vi "Incomplete Analysis.vi"(8 "error constant":errorcluster) -> (0 "error out":errorcluster)   [LabVIEW 2013]
doc: "Use this template to build a simple state machine design pattern. Each state executes code and determines which state to transition to."
uses:
  Analysis Support/Controls/State.ctl
panel:
  out "SPL":dbl
  out "End Flow":dbl format="%0.3f"
  out "Start Flow":dbl format="%0.3f"
  out "Resistance":dbl
  out "Time":dbl
  out "SGP":dbl
  out "selected path":path
  out "Message":string
  in  "Begin":bool
  in  "Exit":bool
  in  "Blank Button":bool
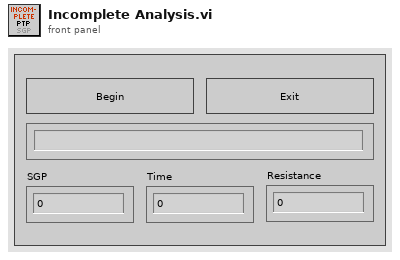
[diagram p1: front panel]
types:
  T1 = typedef "State.ctl" = enum16{"Initialize", "Wait for Event", "Analyze", "Save", "Exit"}
  T2 = enum8{"Enabled", "Disabled", "Disabled and Grayed Out"}
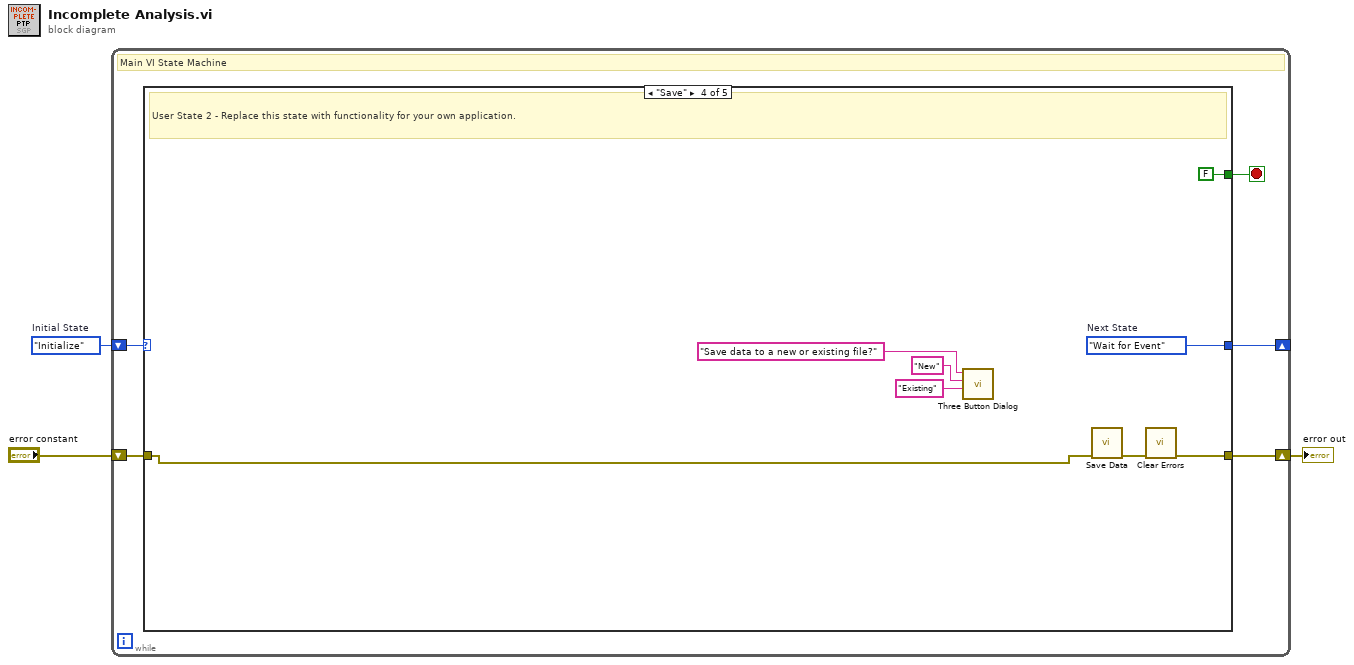
[diagram p0: block diagram]
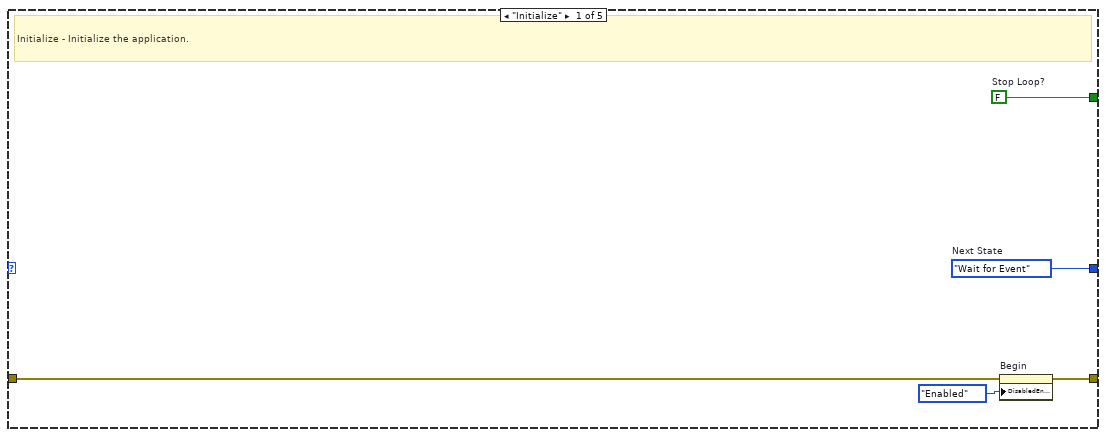
[diagram p2: hidden frame]
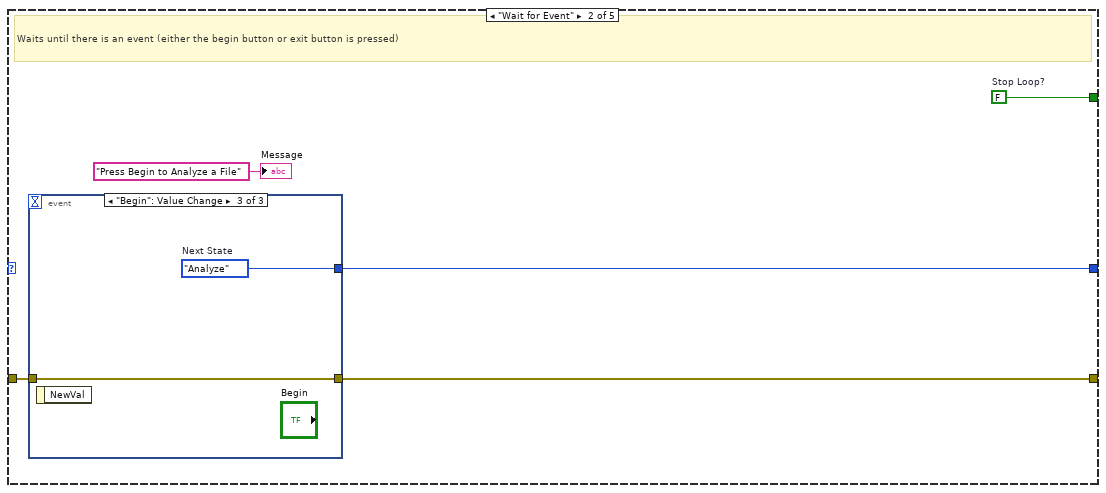
[diagram p3: hidden frame]
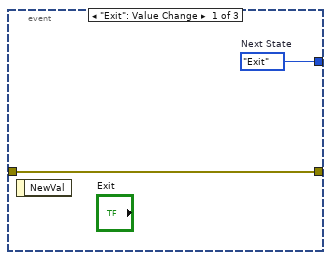
[diagram p4: hidden frame]
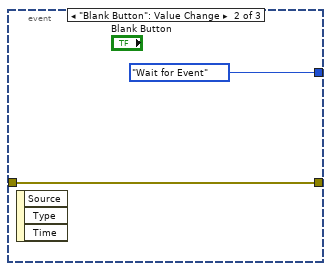
[diagram p5: hidden frame]
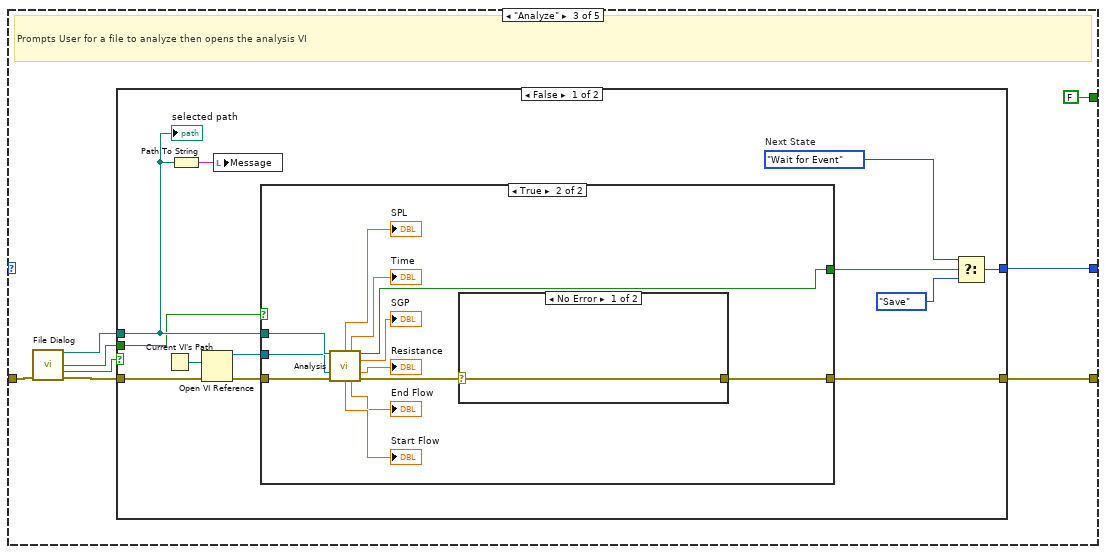
[diagram p6: hidden frame]
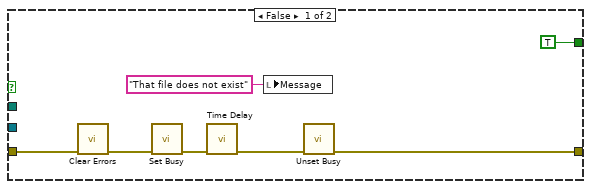
[diagram p7: hidden frame]
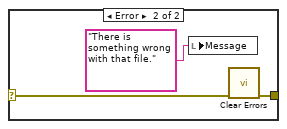
[diagram p8: hidden frame]
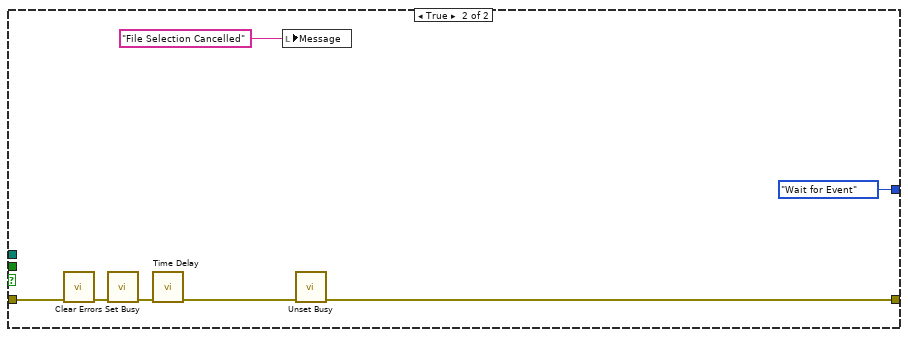
[diagram p9: hidden frame]
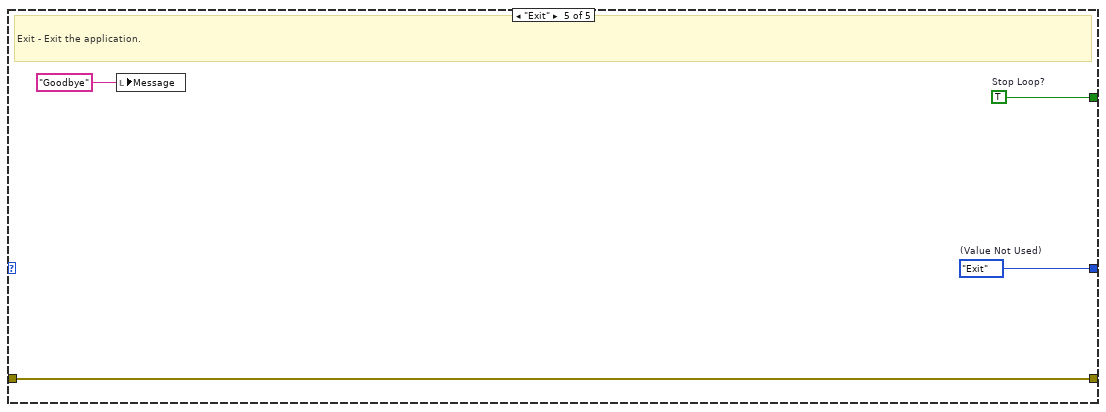
[diagram p10: hidden frame]
diagram:
  w3 = State."Initialize"  # Initial State
  n1 = while {
    shift-right: [w7] -> _
    shift-left: w3 -> [w8]
    shift-right: [w5] -> w1
    shift-left: "error constant" -> [w6]
    stop <- w4 stop-if-true
    # "Main VI State Machine"
    n2 = case shown="\"Save\"" w8 {
      tunnel: [w13 w18 w32 w82 w86] -> w7
      tunnel: [w12 w17 FALSE ("Stop Loop?") FALSE ("Stop Loop?") w85] -> w4
      tunnel: w6 -> [w11 w16 w29 w79 w84]
      tunnel: [w9 w15 w30 w75 w84] -> w5
      frame "Initialize" {
        w12 = FALSE  # Stop Loop?
        w13 = State."Wait for Event"  # Next State
        # "Initialize - Initialize the application."
        n3 = property on="Begin" class="Bool"(error in=w11, "DisabledEnum"=T2."Enabled" ("Disabled")) -> (error out=w9:errorcluster)  [unwired: 1 in, 1 out]
      }
      frame "Wait for Event" {
        w17 = FALSE  # Stop Loop?
        # "Waits until there is an event (either the begin button or exit button is pressed)"
        n4 = event shown="[2] \"Begin\": Value Change" {
          selector: _ -> [_ _ _]
          dyn-events: _ -> [_ _ _]
          timeout: _ -> [_ _ _]
          tunnel: [w20 State."Wait for Event" ("Next State") w24] -> w18
          tunnel: w16 -> [w19 w22 w23]
          tunnel: [w19 w22 w23] -> w15
          event "Exit": Value Change {
            w20 = State."Exit"  # Next State
            n5 = event-data() -> ()  [unwired: 1 in, 1 out]
          }
          event "Blank Button": Value Change {
            n6 = event-data() -> ()  [unwired: 1 in, 3 out]
          }
          event "Begin": Value Change {
            w24 = State."Analyze"  # Next State
            n7 = event-data() -> ()  [unwired: 1 in, 1 out]
          }
        }
        "Message" <- "Press Begin to Analyze a File" ("String")
      }
      frame "Analyze" {
        # "Prompts User for a file to analyze then opens the analysis VI"
        n8 = call "File Dialog"("error in"=w29) -> ("selected path"=w26:path, "exists"=w27:bool, "cancelled"=w25:bool, "error out"=w28:errorcluster)  [unwired: 11 in]
        n9 = case shown="False" w25 {
          tunnel: [w36 State."Wait for Event" ("Next State")] -> w32
          tunnel: [w44 w68] -> w30
          tunnel: w28 -> [w42 w73]
          tunnel: w27 -> [w37 _]
          tunnel: w26 -> [w39 _]
          frame False {
            w35 = State."Wait for Event"  # Next State
            n10 = Current VI's Path() -> (path=w43:path)
            n11 = Path To String(path=w39) -> (string=w38:string)
            n12 = Open VI Reference(vi path=w43, error in (no error)=w42) -> (vi reference=w40:refnum<vi>, error out=w41:errorcluster)  [unwired: 4 in]
            n13 = local write "Message"(w38) -> ()
            n14 = case shown="True" w37 {
              tunnel: [w47 w58] -> w44
              tunnel: w39 -> [_ w63]
              tunnel: w41 -> [w45 w62]
              tunnel: w40 -> [_ w61]
              tunnel: [TRUE ("error?") w60] -> w34
              frame False {
                n15 = call <vilib>:"Clear Errors.vi"("error in (no error)"=w45) -> ("error out"=w46:errorcluster)  [unwired: 6 in]
                n16 = call <vilib>:"Set Busy.vi"("error in (no error)"=w46) -> ("error out"=w49:errorcluster)  [unwired: 9 in, 1 out]
                n17 = call "Time Delay"("error in (no error)"=w49) -> ("error out"=w48:errorcluster)  [unwired: 10 in]
                n18 = local write "Message"("That file does not exist" ("Message")) -> ()
                n19 = call <vilib>:"Unset Busy.vi"("error in (no error)"=w48) -> ("error out"=w47:errorcluster)  [unwired: 10 in]
              }
              frame True {
                n20 = call "Analysis.vi"("selected path"=w63, "VI reference"=w61, "error in (no error)"=w62) -> ("SPL"=→"SPL":dbl, "Interruption Time (Out)"=→"Time":dbl, "error?"=w60:bool, "SGP"=→"SGP":dbl, "Resistance (Out)"=→"Resistance":dbl, "Start Flow"=→"Start Flow":dbl, "End Flow"=→"End Flow":dbl, "error out"=w59:errorcluster)  [unwired: 5 in]
                n21 = case shown="No Error" w59 {
                  selector: w59 -> [w64 w66]
                  tunnel: [w64 w65] -> w58
                  frame No Error {
                  }
                  frame Error {
                    n22 = local write "Message"("There is something wrong with that file." ("Message")) -> ()
                    n23 = call <vilib>:"Clear Errors.vi"("error in (no error)"=w66) -> ("error out"=w65:errorcluster)  [unwired: 6 in]
                  }
                }
              }
            }
            n24 = Select(t=w35, s=w34, f=State."Save") -> (s? t:f=w36:T1)
            "selected path" <- w39
          }
          frame True {
            n25 = call <vilib>:"Clear Errors.vi"("error in (no error)"=w73) -> ("error out"=w70:errorcluster)  [unwired: 6 in]
            n26 = call <vilib>:"Set Busy.vi"("error in (no error)"=w70) -> ("error out"=w71:errorcluster)  [unwired: 9 in, 1 out]
            n27 = call "Time Delay"("error in (no error)"=w71) -> ("error out"=w69:errorcluster)  [unwired: 10 in]
            n28 = local write "Message"("File Selection Cancelled" ("Message")) -> ()
            n29 = call <vilib>:"Unset Busy.vi"("error in (no error)"=w69) -> ("error out"=w68:errorcluster)  [unwired: 10 in]
          }
        }
      }
      frame "Save" {
        w82 = State."Wait for Event"  # Next State
        # "User State 2 - Replace this state with functionality for your own application."
        n30 = call <vilib>:"Three Button Dialog.vi"("Center Button Text (\"No\")"="Existing" ("T button name (\"OK\")"), "Left Button Text (\"Yes\")"="New" ("F button name (\"Cancel\")"), "message"="Save data to a new or existing file?") -> ()  [unwired: 8 in, 1 out]
        n31 = call "Save Data.vi"("error in (no error)"=w79) -> ("error out"=w76:errorcluster)  [unwired: 14 in]
        n32 = call <vilib>:"Clear Errors.vi"("error in (no error)"=w76) -> ("error out"=w75:errorcluster)  [unwired: 6 in]
      }
      frame "Exit" {
        w85 = TRUE  # Stop Loop?
        w86 = State."Exit"  # (Value Not Used)
        # "Exit - Exit the application."
        n33 = local write "Message"("Goodbye" ("Message")) -> ()
      }
    }
  }
  "error out" <- w1
